vi "worksheet filter column.vi"(8 "error in (no error)":errorcluster, 9 "rule":u32, 10 "col":u16, 11 "worksheet":u32) -> (0 "error out":errorcluster, 3 "function return":u32(ring))   [LabVIEW 8.6]
doc: "lxw_error worksheet_filter_column(lxw_worksheet worksheet, lxw_col_t col, unsigned long rule);"
uses:
  pending_lvxlsxwriter/xlsxwriter.dll
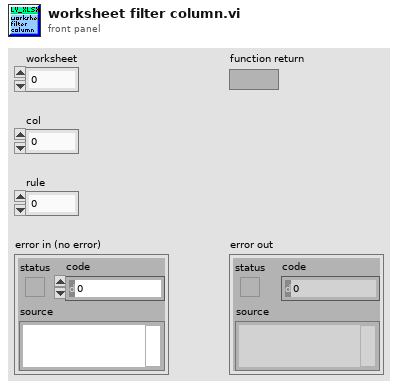
[diagram p1: front panel]
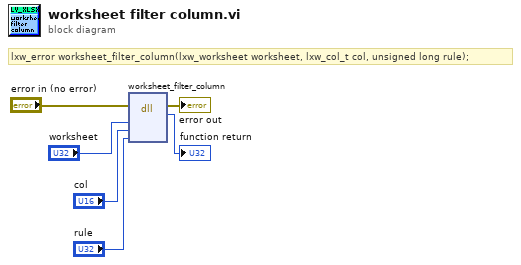
[diagram p0: block diagram]
diagram:
  # "lxw_error worksheet_filter_column(lxw_worksheet worksheet, lxw_col_t col, unsigned long rule);"
  n1 = dll-call lib="C:/Users/WDAGUtilityAccount/Desktop/pending_lvxlsxwriter/xlsxwriter.*" fn="worksheet_filter_column"(error in="error in (no error)", "worksheet"="worksheet", "col"="col", "rule"="rule") -> (error out=→"error out":errorcluster, →"function return":u32)  [unwired: 5 in, 1 out]
